vi "Circular Buffer Waveforms.vi"(6 "Action":T1, 8 "Error In":errorcluster, 9 "New Data":waveform(dbl)[](array[waveform]), 10 "Size":i32) -> (0 "Error Out":errorcluster, 1 "Buffer Out":waveform(dbl)[][](array[waveform]), 2 "Iterations":i32, 5 "Ready":bool)   [LabVIEW 2016]
uses:
  Circular Buffer Operations.ctl
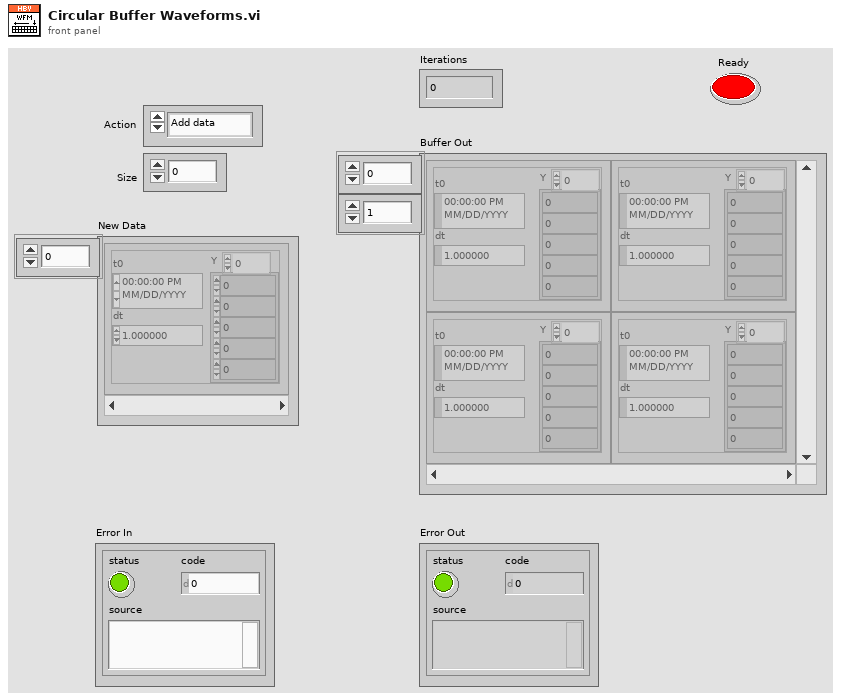
[diagram p1: front panel]
types:
  T1 = typedef "Circular Buffer Operations.ctl" = enum16{"Add data", "Reset"}
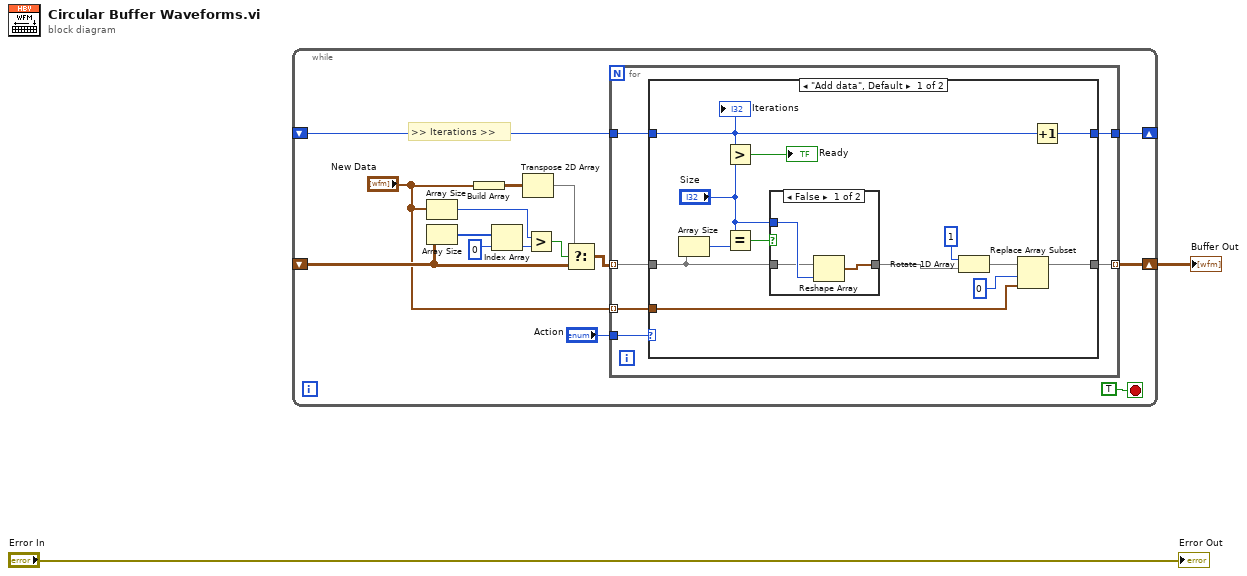
[diagram p0: block diagram]
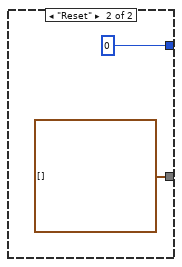
[diagram p3: hidden frame]
diagram:
  n1 = while {
    shift-right: [w17] -> w2
    shift-left: _ -> [w12]
    shift-right: [w14] -> _
    shift-left: _ -> [w13]
    stop <- TRUE stop-if-true
    # ">> Iterations >>"
    n2 = Array Size(array="New Data") -> (size(s)=w5:i32)
    n3 = Array Size(array=w12) -> (size(s)=w7:i32[])
    n4 = Build Array("New Data") -> (w9:waveform(dbl)[][])
    n5 = Index Array(array=w7, index=0) -> (element=w4:i32)
    n6 = Transpose 2D Array(2D array=w9) -> (transposed array=w10:waveform(dbl)[][])
    n7 = Greater?(x=w5, y=w4) -> (0:w3:bool)
    n8 = Select(t=w10, s=w3, f=w12) -> (s? t:f=w11:waveform(dbl)[][])
    n9 = for {
      tunnel: [w23] -> w17 mode=indexing
      tunnel: w11 -> [w22] mode=indexing
      tunnel: "Action" -> [w21]
      tunnel: [w20] -> w14
      tunnel: w13 -> [w19]
      tunnel: "New Data" -> [w18] mode=indexing
      n10 = case shown="\"Add data\", Default" w21 {
        tunnel: [w33 waveform(dbl)[] []] -> w23
        tunnel: w22 -> [w27 _]
        tunnel: [w32 0] -> w20
        tunnel: w19 -> [w31 _]
        tunnel: w18 -> [w24 _]
        frame "Add data", Default {
          n11 = Array Size(array=w27) -> (size(s)=w29:i32)
          n12 = Greater?(x=w31, y="Size") -> (0:→"Ready":bool)
          n13 = Equal?(x="Size", y=w29) -> (x = y?=w28:bool)
          n14 = case shown="False" w28 {
            tunnel: "Size" -> [w39 _]
            tunnel: w27 -> [w38 w40]
            tunnel: [w37 w40] -> w26
            frame False {
              n15 = Reshape Array(w38, w39) -> (w37:waveform(dbl)[])
            }
            frame True {
            }
          }
          n16 = Rotate 1D Array(1:w26, 2:1 ("n")) -> (0:w34:waveform(dbl)[])
          n17 = Replace Array Subset(array=w34, new element=w24, index=0) -> (w33:waveform(dbl)[])
          n18 = Increment(x=w31) -> (x+1=w32:i32)
          "Iterations" <- w31
        }
        frame "Reset" {
        }
      }
    }
  }
  "Buffer Out" <- w2
  "Error Out" <- "Error In"
